vi "Using Connection Strings.vi"() -> ()   [LabVIEW 2018]
doc: "This example shows how to build an executable that uses the Database Connectivity Toolkit. It also shows how to dynamically create a connection string so the database being used can move with the executable."
uses:
  <vilib>/addons/database/Auxilliary.llb/DB Tools Cursor Type.ctl
  <vilib>/addons/database/Connection.llb/DB Tools Open Connec (String).vi
  <vilib>/addons/database/Connection.llb/Conn Execute.vi
  <vilib>/addons/database/Recordset.llb/Rec Get Recordset Properties (R).vi
  <vilib>/addons/database/Recordset.llb/Rec Move To Record N (R).vi
  <vilib>/addons/database/Recordset.llb/Rec Fetch Recordset Data (R).vi
  <vilib>/addons/database/Recordset.llb/Rec Destroy - Connection.vi
  <vilib>/addons/database/_DB Variant To Data/Database Variant To Data.xnode
  <vilib>/addons/database/NI_Database_API.lvlib
panel:
  out "String read from database":string
  out "Numeric read from database":i32
  out "Date/Time read from database":timestamp
  in  "String to insert":string="this is a test."
  in  "Numeric to insert":i32=125
  out "Date/Time inserted":timestamp
  # "Overview: Demonstrates the functionality of the Database Connectivity Toolkit in a LabVIEW built executable.\nRequirements: Database Connectivity Toolkit, LabVIEW Professional Development System or LabVIEW Application Builder\nInstructions:\n1. In the 'Using Connection Strings.lvproj' that owns this VI, expand the Build Specifications item.\n2. Right-click Connecting to a database in an EXE and select Build.\n3. When the build is complete, click Done.\n4. Right-click 'Connecting to a database in an EXE' and select Run to run the built executable that calls Database Toolkit VIs."
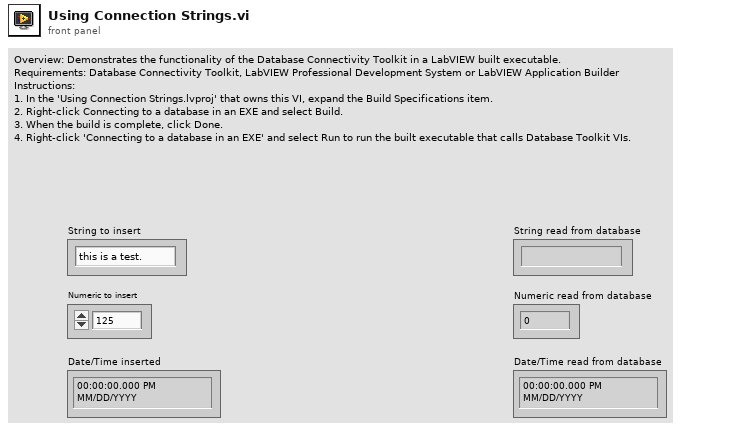
[diagram p1: front panel]
types:
  T1 = typedef "NI_Database_API.lvlib/DB Tools Cursor Type.ctl" = enum16{"forward-only", "keyset", "dynamic", "static"}
  T2 = enum32{"invalid app kind", "Development System", "Run Time System", "Student Edition", "Embedded LabVIEW", "Evaluation", "Custom"}
  T3 = typedef "NI_Database_API.lvlib/Conn ObjectReference.ctl" = refnum<k1>
  T4 = cluster{"String to insert":string, "Numeric to insert":i32, "seconds since 1Jan1904":timestamp}
  T5 = typedef "NI_Database_API.lvlib/Rec ObjectReference.ctl" = refnum<k1>
  T6 = typedef "NI_Database_API.lvlib/Rec Properties.ctl" = cluster{"column count":i32, "record index":i32, "record count":i32, "bof?":bool, "eof?":bool, "cursor type":T1, "cache size":i32, "state":enum16{"closed", "open"}}
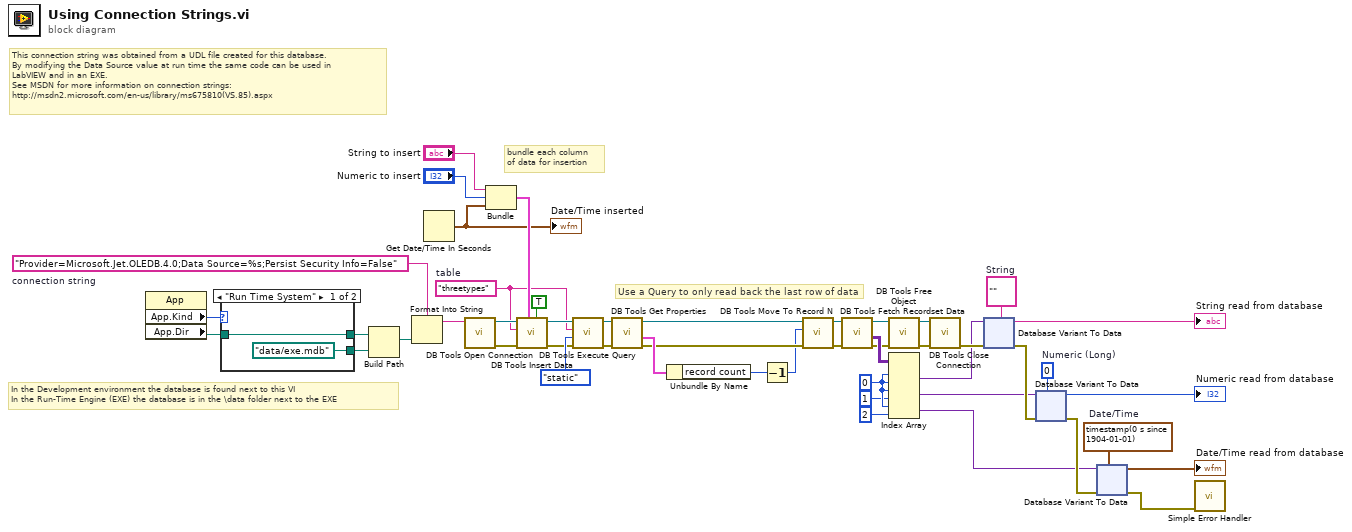
[diagram p0: block diagram]
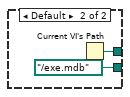
[diagram p2: hidden frame]
diagram:
  w1 = "Provider=Microsoft.Jet.OLEDB.4.0;Data Source=%s;Persist Security Info=False"  # connection string
  w2 = "threetypes"  # table
  w3 = ""  # String
  w4 = 0  # Numeric (Long)
  w7 = 0 ("disabled index (col)")
  w37 = timestamp(0 s since 1904-01-01)  # Date/Time
  # "This connection string was obtained from a UDL file created for this database.\nBy modifying the Data Source value at run time the same code can be used in\nLabVIEW and in an EXE.\nSee MSDN for more information on connection strings:\nhttp://msdn2.microsoft.com/en-us/library/ms675810(VS.85).aspx"
  # "In the Development environment the database is found next to this VI\nIn the Run-Time Engine (EXE) the database is in the \\data folder next to the EXE"
  # "Use a Query to only read back the last row of data"
  # "bundle each column\nof data for insertion"
  n1 = property class="App"() -> ("App.Kind"=w35:T2, "App.Dir"=w34:path)  [unwired: 2 in, 2 out]
  n2 = case shown="\"Run Time System\"" w35 {
    tunnel: w34 -> [w50 _]
    tunnel: [path "data/exe.mdb" ("path") path "../exe.mdb" ("path")] -> w32
    tunnel: [w50 w51] -> w31
    frame "Run Time System" {
    }
    frame Default {
      n3 = Current VI's Path() -> (path=w51:path)
    }
  }
  n4 = Build Path(base path=w31, name or relative path=w32) -> (appended path=w33:path)
  n5 = Format Into String(format string=w1, w33) -> (resulting string=w38:string)  [unwired: 2 in, 1 out]
  n6 = Get Date/Time In Seconds() -> (seconds since 1Jan1904=w36:timestamp)
  "Date/Time inserted" <- w36
  n7 = call-poly <vilib>:"DB Tools Open Connection.vi"("connection information"=w38) -> ("error out"=w28:errorcluster, "connection reference"=w29:T3)  [unwired: 7 in]
  n8 = Bundle("String to insert"="String to insert", "Numeric to insert"="Numeric to insert", "seconds since 1Jan1904"=w36) -> (w48:T4)  [unwired: 1 in]
  n9 = call <vilib>:"DB Tools Insert Data.vi"("create table? (F)"=TRUE ("create table? (f)"), "data"=w48, "error in (no error)"=w28, "table"=w2, "connection reference"=w29) -> ("error out"=w11:errorcluster, "connection reference out"=w12:T3)  [unwired: 5 in]
  n10 = call-poly <vilib>:"DB Tools Execute Query.vi"("error in (no error)"=w11, "cursor type"=DB_Tools_Cursor_Type."static", "SQL query"=w2, "connection reference"=w12) -> ("error out"=w25:errorcluster, "recordset reference"=w26:T5)  [unwired: 4 in]
  n11 = call-poly <vilib>:"DB Tools Get Properties.vi"("error in (no error)"=w25, "recordset reference"=w26) -> ("error out"=w21:errorcluster, "recordset properties"=w24:T6, "recordset reference out"=w22:T5)  [unwired: 3 in]
  n12 = Unbundle By Name(w24) -> ("record count"=w23:i32)
  n13 = Decrement(x=w23) -> (x-1=w13:i32)
  n14 = call-poly <vilib>:"DB Tools Move To Record N.vi"("error in (no error)"=w21, "n (0)"=w13, "recordset reference"=w22) -> ("error out"=w20:errorcluster, "recordset reference out"=w19:T5)  [unwired: 7 in]
  n15 = call-poly <vilib>:"DB Tools Fetch Recordset Data.vi"("error in (no error)"=w20, "recordset reference"=w19) -> ("error out"=w15:errorcluster, "recordset data"=w18:variant[][], "recordset reference out"=w17:T5)  [unwired: 3 in]
  n16 = call-poly <vilib>:"DB Tools Free Object.vi"("error in (no error)"=w15, "recordset reference"=w17) -> ("error out"=w14:errorcluster, "connection reference"=w16:T3)  [unwired: 8 in]
  n17 = Index Array(array=w18, index (row) #1=w7, index (col) #1=w7, index (row) #2=w7, index (col) #2=1 ("disabled index (col)"), index (row) #3=w7, index (col) #3=2 ("disabled index (col)")) -> (element #1=w10:variant, element #2=w9:variant, element #3=w8:variant)
  n18 = call <vilib>:"DB Tools Close Connection.vi"("error in (no error)"=w14, "connection reference"=w16) -> ("error out"=w45:errorcluster)  [unwired: 5 in]
  n19 = xnode "Database Variant To Data"("database variant"=w10, "error in (no error)"=w45, "type"=w3) -> ("data"=→"String read from database":string, "error out"=w41:errorcluster)
  n20 = xnode "Database Variant To Data"("database variant"=w9, "error in (no error)"=w41, "type"=w4) -> ("data"=→"Numeric read from database":i32, "error out"=w39:errorcluster)
  n21 = xnode "Database Variant To Data"("database variant"=w8, "error in (no error)"=w39, "type"=w37) -> ("data"=→"Date/Time read from database":timestamp, "error out"=w40:errorcluster)
  n22 = call <vilib>:"Simple Error Handler.vi"("error in (no error)"=w40) -> ()  [unwired: 4 in, 5 out]
